vi "SVT Max Frequency Within Tolerances.vi"(8 "error in (no error)":errorcluster, 9 "type":enum16{"Type 0", "Type 1"}(ring), 10 "weighting":u16(ring) items=["Linear", "A-weighting", "B-weighting", "C-weighting"], 11 "sampling frequency [Hz]":dbl=51200.0 format="%.2f") -> (0 "error out":errorcluster, 3 "max freq within tolerances [Hz]":dbl format="%.2f")   [LabVIEW 2017, in "SoundVib_ABCWeighting.lvlib"]
doc: "Returns the maximum frequency within tolerances according to the ANSI S1.4 standard and based on <B>sampling frequency [Hz]</B>, <B>weighting</B>, and <B>type</B>."
uses:
  <vilib>/addons/Sound and Vibration/svt_Weighting/SoundVib_ABCWeighting.lvlib
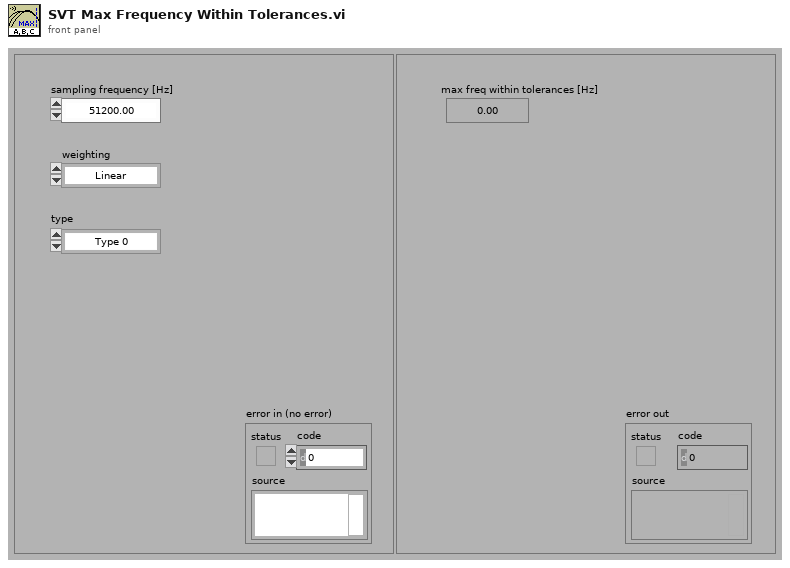
[diagram p1: front panel]
types:
  T1 = cluster{"filter structure":enum32{"IIR 2nd Order", "IIR 4th Order"}, "Reverse Coefficients":dbl[], "Forward Coefficients":dbl[]}
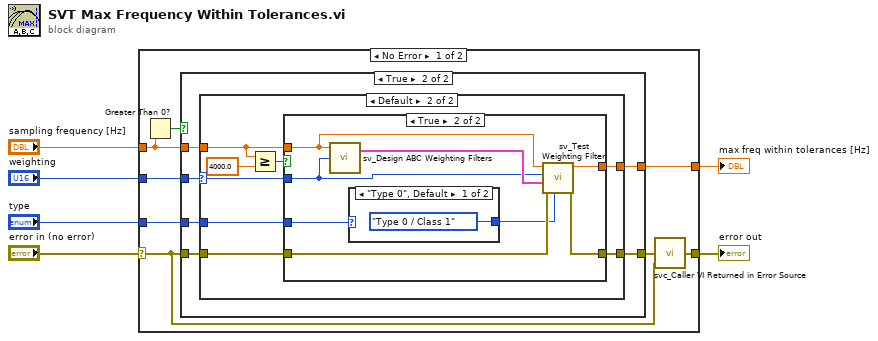
[diagram p0: block diagram]
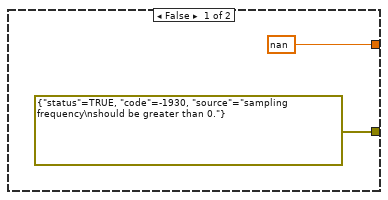
[diagram p2: hidden frame]
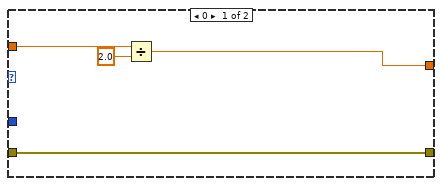
[diagram p3: hidden frame]
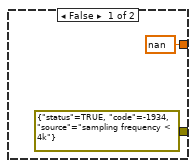
[diagram p4: hidden frame]
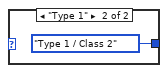
[diagram p5: hidden frame]
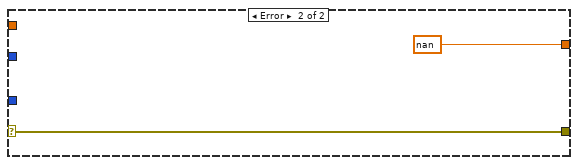
[diagram p6: hidden frame]
diagram:
  n1 = case shown="No Error" "error in (no error)" {
    selector: "error in (no error)" -> [w7 w48]
    tunnel: [w12 w48] -> w5
    tunnel: "weighting" -> [w14 _]
    tunnel: [w13 nan] -> w3
    tunnel: "sampling frequency [Hz]" -> [w8 _]
    tunnel: "type" -> [w11 _]
    frame No Error {
      n2 = Greater Than 0?(x=w8) -> (x > 0?=w10:bool)
      n3 = case shown="True" w10 {
        tunnel: w14 -> [_ w17]
        tunnel: [nan ("max freq within tolerances [Hz]") w22] -> w13
        tunnel: w8 -> [_ w20]
        tunnel: w11 -> [_ w21]
        tunnel: w7 -> [_ w19]
        tunnel: [errorcluster {"status"=TRUE, "code"=-1930, "source"="sampling frequency\nshould be greater than 0."} ("error in (no error)") w18] -> w9
        frame False {
        }
        frame True {
          n4 = case shown="Default" w17 {
            selector: w17 -> [_ w27]
            tunnel: [w24 w34] -> w22
            tunnel: w21 -> [_ w33]
            tunnel: w20 -> [w26 w32]
            tunnel: w19 -> [w23 w29]
            tunnel: [w23 w28] -> w18
            frame 0 {
              n5 = Divide(x=w26, y=2.0) -> (x/y=w24:dbl)
            }
            frame Default {
              n6 = Greater Or Equal?(x=w32, y=4000.0) -> (x >= y?=w30:bool)
              n7 = case shown="True" w30 {
                tunnel: w27 -> [_ w38]
                tunnel: [nan ("max freq within tolerances [Hz]") w42] -> w34
                tunnel: w32 -> [_ w37]
                tunnel: w33 -> [_ w40]
                tunnel: w29 -> [_ w44]
                tunnel: [errorcluster {"status"=TRUE, "code"=-1934, "source"="sampling frequency < 4k"} ("error out") w43] -> w28
                frame False {
                }
                frame True {
                  n8 = call <vilib>:"sv_Design ABC Weighting Filters.vi"("weighting"=w38, "sampling frequency [Hz]"=w37) -> ("filter coefficients"=w41:T1)  [unwired: 2 in]
                  n9 = case shown="\"Type 0\", Default" w40 {
                    tunnel: [enum16{"Type 0 / Class 1", "Type 1 / Class 2"}."Type 0 / Class 1" ("type or class") enum16{"Type 0 / Class 1", "Type 1 / Class 2"}."Type 1 / Class 2" ("type or class")] -> w39
                    frame "Type 0", Default {
                    }
                    frame "Type 1" {
                    }
                  }
                  n10 = call <vilib>:"sv_Test Weighting Filter.vi"("type or class"=w39, "error in (no error)"=w44, "filter coefficients"=w41, "weighting"=w38, "sampling frequency [Hz]"=w37) -> ("error out"=w43:errorcluster, "max freq within tolerances [Hz]"=w42:dbl)  [unwired: 5 in]
                }
              }
            }
          }
        }
      }
      n11 = call <vilib>:"svc_Caller VI Returned in Error Source.vi"("warning input to caller"=w7, "error in (no error)"=w9) -> ("error out"=w12:errorcluster)  [unwired: 3 in]
    }
    frame Error {
    }
  }
  "error out" <- w5
  "max freq within tolerances [Hz]" <- w3
